vi "pdv_usb1.vi"() -> ()   [LabVIEW 2010]
uses:
  70user.lib/TheSigTab.vi
  <vilib>/Utility/config.llb/Read Key (U32).vi
  <vilib>/addons/database/Connection.llb/DB Tools Open Connec (Path).vi
  <vilib>/Utility/config.llb/Read Key (String).vi
  <vilib>/Utility/config.llb/Write Key (Double).vi
  <vilib>/Utility/config.llb/Write Key (U32).vi
  <vilib>/addons/database/NI_Database_API.lvlib
  <vilib>/Utility/config.llb/NI_LVConfig.lvlib
panel:
  in  "ScopeToo":bool caption="Сохранять осциллограммы"
  in  "m_s":u16(ring) items=["мин", "сек"]
  in  "Object":string(combo) caption="Объект"
  in  "CurvesToo":bool caption="Сохранять графики"
  in  "AcqureTime":dbl caption="опроса" format="%#.3g"
  out "ExtDev":bool caption="Выносной модуль"
  in  "SaveTime":dbl=1.0 caption="мин" min=1.0 max=120.0
  out "Slide":u8(slide) scale=0.0..100.0
  in  "Continuosly":bool caption="Периодически"
  in  "SaveNow":bool caption="Однократно"
  in  "Loop":bool caption="Зациклить данные"
  out "Current time":timestamp caption="Время и Дата" format="%<%X\n%x>T"
  out "Tper":dbl caption="общая"
  in  "filter":bool caption="Фильтр\nперекрёстных помех"
  in  "Stop":bool
  in  "Table":string[][](table) caption="Результаты измерений"
  # "Запись в базу данных"
  # "Продолжительность, с"
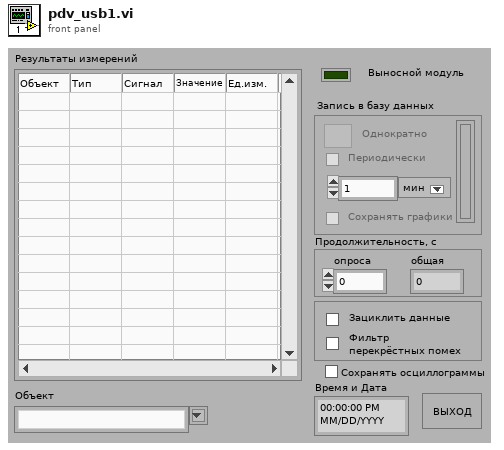
[diagram p1: front panel]
types:
  T1 = typedef "NI_LVConfig.lvlib/Config Data RefNum.ctl" = refnum<k1>
  T2 = typedef "NI_Database_API.lvlib/Conn ObjectReference.ctl" = refnum<k1>
  T3 = cluster{"Status":bool, "ViErrorNumber":u32, "ViName":string, "ViErrorString":string, "CinName":string, "CinErrorString":string}
  T4 = cluster{"VirtualSlot":u16, "ModuleName":string, "SerialNumber":string, "UsbSpeed":u8, "AvrVersion":string, "ModuleRevision":string, "DspType":string, "IsDacPresented":bool, "DspLoading":bool, "DspVersion":string, "DspClockout":u32, "AdcOffsetCoef":sgl[], "AdcScaleCoef":sgl[], "DacOffsetCoef":sgl[], "DacScaleCoef":sgl[]}
  T5 = cluster{"DllVersion":u32, "InterfaceType":u32, "InterfaceInstance":u32, "ModuleHandle":u32, "ReadBuffersParsArray":cluster{"Buffer":i16[], "ReadOv":u32, "ReadEvent":u32}[], "WriteBuffersParsArray":cluster{"Buffer":i16[], "WriteOv":u32, "WriteEvent":u32}[]}
  T6 = cluster{"Сигнал":string, "Тип":enum16{"Напряжение/Ток", "ЧР", "Температура", "Давление"}, "Object":string}[]
  T7 = cluster{"Сигнал":string, "Тип":enum16{"Напряжение/Ток", "ЧР", "Температура", "Давление"}, "Object":string}
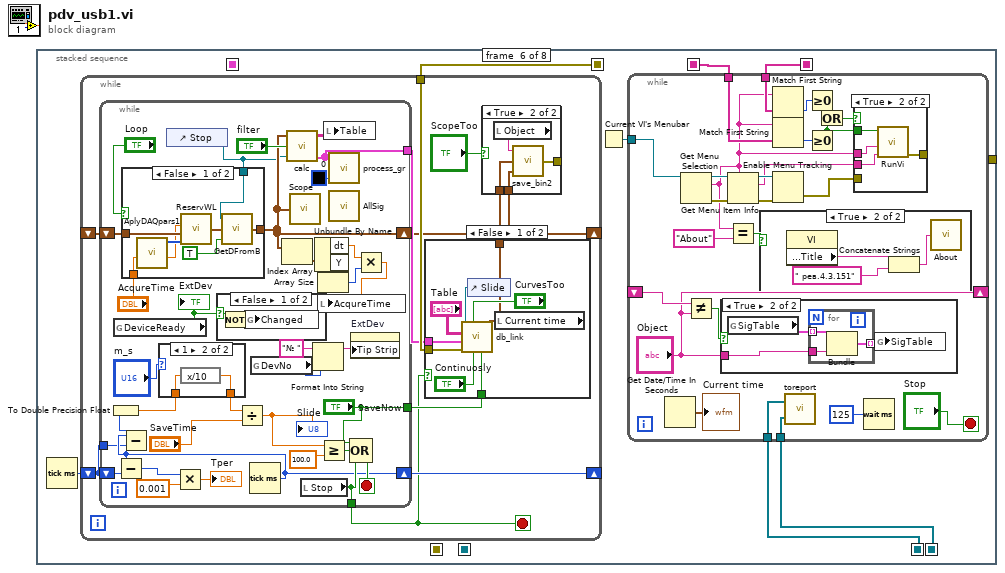
[diagram p0: block diagram]
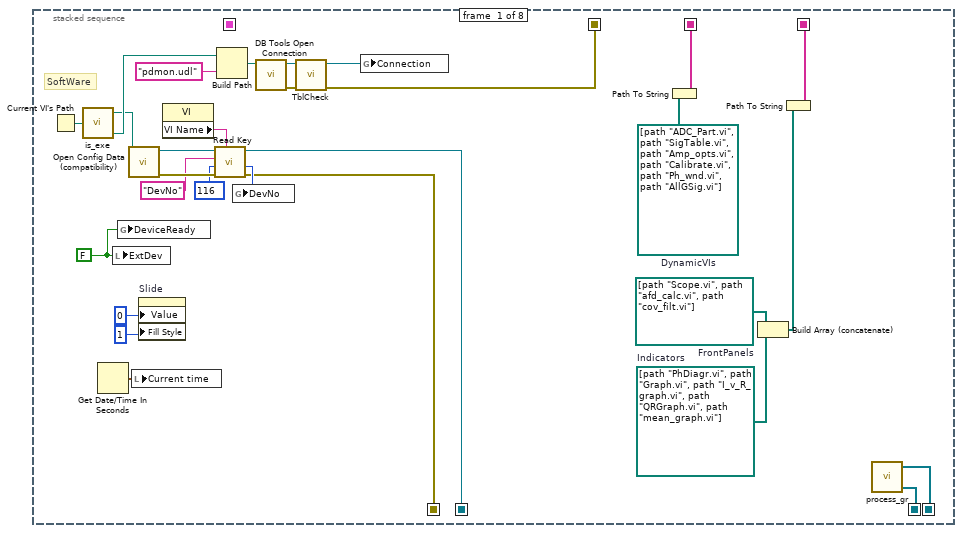
[diagram p2: hidden frame]
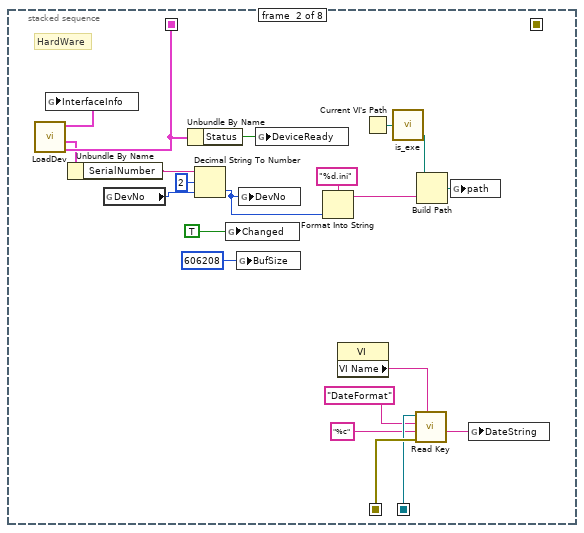
[diagram p3: hidden frame]
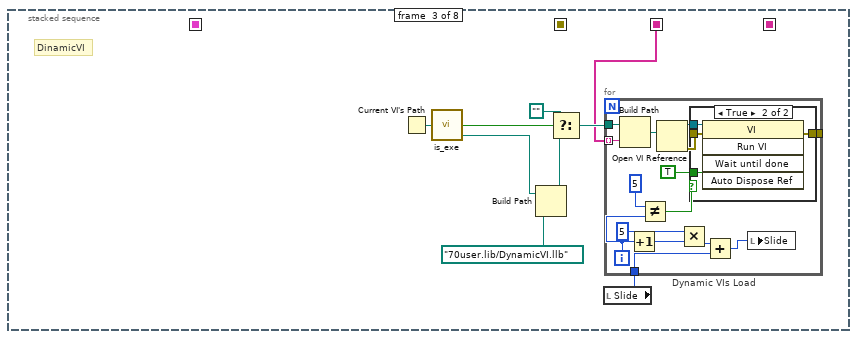
[diagram p4: hidden frame]
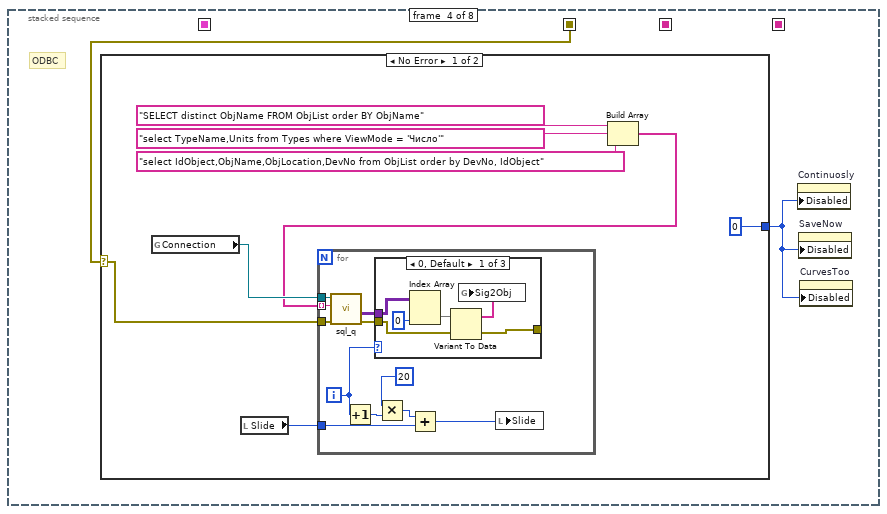
[diagram p6: hidden frame]
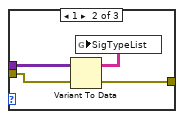
[diagram p7: hidden frame]
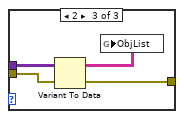
[diagram p8: hidden frame]
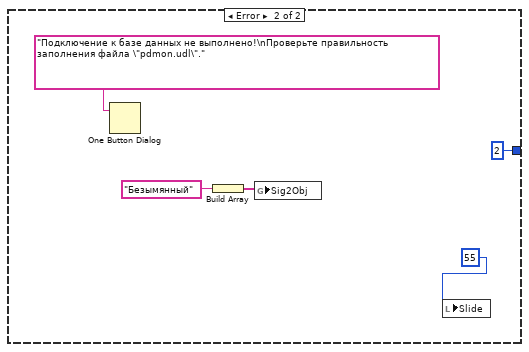
[diagram p9: hidden frame]
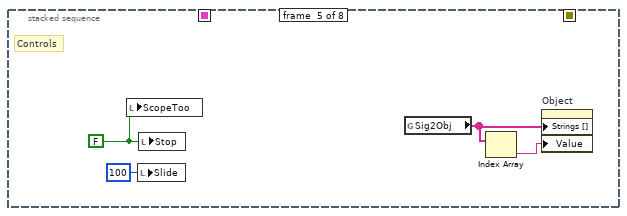
[diagram p10: hidden frame]
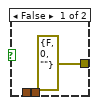
[diagram p11: hidden frame]
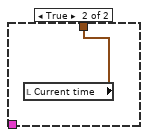
[diagram p12: hidden frame]
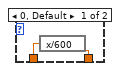
[diagram p13: hidden frame]
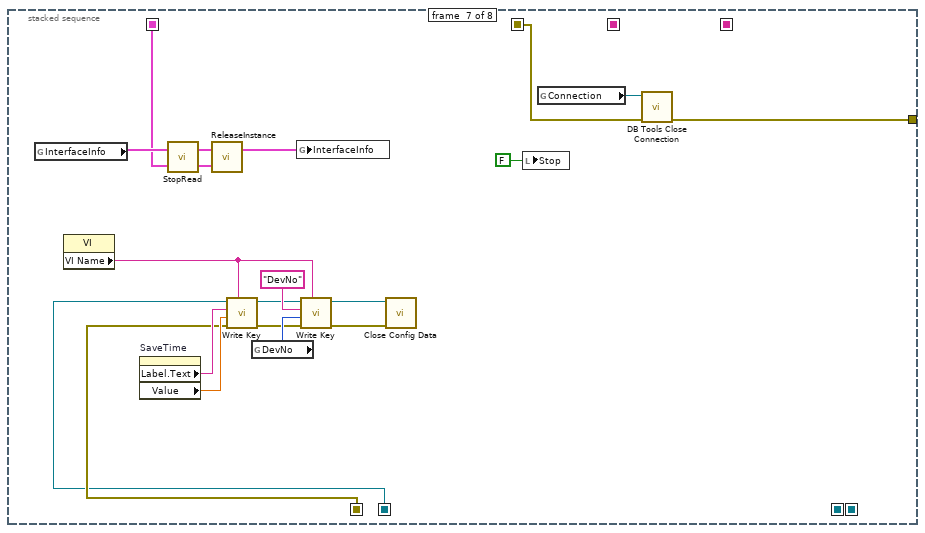
[diagram p19: hidden frame]
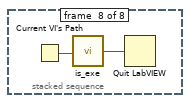
[diagram p20: hidden frame]
diagram:
  n1 = stacked-sequence {
    seq-local: [_ w45 _ _ _ _ _ _] -> [_ _ _ _ _ _ w256 _]
    seq-local: [w15 _ _ _ _ _ _ _] -> [_ _ _ w81 _ w129 w263 _]
    seq-local: [w18 _ _ _ _ _ _ _] -> [_ _ _ _ _ w127 _ _]
    seq-local: [w22 _ _ _ _ _ _ _] -> [_ _ w54 _ _ w126 _ _]
    seq-local: [w25 _ _ _ _ _ _ _] -> [_ _ _ _ _ w124 _ _]
    seq-local: [w24 _ _ _ _ _ _ _] -> [_ _ _ _ _ w125 _ _]
    seq-local: [w2 _ _ _ _ _ _ _] -> [_ w34 _ _ _ _ w244 _]
    seq-local: [w1 _ _ _ _ _ _ _] -> [_ w35 _ _ _ _ w245 _]
    tunnel: [_ _ _ _ _ _ w260 _] -> _
    frame #0 {
      w4 = FALSE ("ExtDev")
      w20 = path[] [path "PhDiagr.vi", path "Graph.vi", path "I_v_R_graph.vi", path "QRGraph.vi", path "mean_graph.vi"]  # Indicators
      w21 = path[] [path "Scope.vi", path "afd_calc.vi", path "cov_filt.vi"]  # FrontPanels
      w23 = path[] [path "ADC_Part.vi", path "SigTable.vi", path "Amp_opts.vi", path "Calibrate.vi", path "Ph_wnd.vi", path "AllGSig.vi"]  # DynamicVIs
      # "SoftWare"
      n2 = Current VI's Path() -> (path=w29:path)
      n3 = call "is_exe.vi"("path"=w29) -> ("actual path"=w28:path, "ini path"=w10:path)  [unwired: 2 in, 1 out]
      n4 = Get Date/Time In Seconds() -> (seconds since 1Jan1904=w13:timestamp)
      n5 = local write "ExtDev"(w4) -> ()
      n6 = global write "TheSigTab.vi" "DeviceReady"(w4) -> ()
      n7 = call <vilib>:"Open Config Data (compatibility).vi"("configuration file path"=w10) -> ("error out"=w8:errorcluster, "refnum"=w9:T1)  [unwired: 8 in, 1 out]
      n8 = local write "Current time"(w13) -> ()
      n9 = property on="Slide" class="Slide (strict)"("Value"=u8 0 ("Slide"), "Fill Style"=1) -> ()  [unwired: 2 in, 2 out]
      n10 = property class="VI"() -> ("VI Name"=w3:string)  [unwired: 2 in, 2 out]
      n11 = call-poly <vilib>:"Read Key.vi"("section"=w3, "error in (no error)"=w8, "default value"=u32 116 ("DevNo"), "key"="DevNo", "refnum"=w9) -> ("error out"=w1:errorcluster, "value"=w5:u32, "refnum out"=w2:T1)  [unwired: 3 in, 1 out]
      n12 = Build Path(base path=w28, name or relative path="pdmon.udl") -> (appended path=w26:path)
      n13 = global write "TheSigTab.vi" "DevNo"(w5) -> ()
      n14 = call-poly <vilib>:"DB Tools Open Connection.vi"("connection information"=w26) -> ("error out"=w16:errorcluster, "connection reference"=w17:T2)  [unwired: 7 in]
      n15 = call "TblCheck.vi"("error in"=w16, "connection reference"=w17) -> ("error out"=w15:errorcluster, "conn ref out"=w14:T2)  [unwired: 3 in, 1 out]
      n16 = global write "TheSigTab.vi" "Connection"(w14) -> ()
      n17 = Path To String(path=w23) -> (string=w22:string[])
      n18 = Build Array (concatenate)(w21, w20) -> (w19:path[])
      n19 = Path To String(path=w19) -> (string=w18:string[])
      n20 = call "process_gr.vi"() -> ("WG refs"=w25:refnum<vi>[], "menu refs"=w24:refnum<k9>[])  [unwired: 4 in]
    }
    frame #1 {
      # "HardWare"
      n21 = call "LoadDev.vi"() -> ("ViStatus"=w45:T3, "ModuleInfo"=w44:T4, "InterfaceInfo"=w46:T5)  [unwired: 5 in]
      n22 = global write "TheSigTab.vi" "InterfaceInfo"(w46) -> ()
      n23 = Unbundle By Name(w44) -> ("SerialNumber"=w43:string)
      n24 = global read "TheSigTab.vi" "DevNo"() -> (w36:u32)
      n25 = Unbundle By Name(w45) -> ("Status"=w50:bool)
      n26 = Decimal String To Number(string=w43, offset=u32 2 ("initial scan location"), default (0L)=w36) -> (number=w38:u32)  [unwired: 1 out]
      n27 = global write "TheSigTab.vi" "Changed"(TRUE ("Changed")) -> ()
      n28 = global write "TheSigTab.vi" "BufSize"(u32 606208 ("BufSize")) -> ()
      n29 = global write "TheSigTab.vi" "DevNo"(w38) -> ()
      n30 = global write "TheSigTab.vi" "DeviceReady"(w50) -> ()
      n31 = Format Into String(format string="%d.ini", w38) -> (resulting string=w40:string)  [unwired: 2 in, 1 out]
      n32 = property class="VI"() -> ("VI Name"=w33:string)  [unwired: 2 in, 2 out]
      n33 = Current VI's Path() -> (path=w49:path)
      n34 = call "is_exe.vi"("path"=w49) -> ("actual path"=w37:path)  [unwired: 2 in, 2 out]
      n35 = call-poly <vilib>:"Read Key.vi"("section"=w33, "error in (no error)"=w35, "default value"="%c", "key"="DateFormat", "refnum"=w34) -> ("value"=w30:string)  [unwired: 3 in, 3 out]
      n36 = Build Path(base path=w37, name or relative path=w40) -> (appended path=w39:path)
      n37 = global write "TheSigTab.vi" "path"(w39) -> ()
      n38 = global write "TheSigTab.vi" "DateString"(w30) -> ()
    }
    frame #2 {
      # "DinamicVI"
      n39 = Current VI's Path() -> (path=w53:path)
      n40 = call "is_exe.vi"("path"=w53) -> ("actual path"=w51:path, "exe?"=w52:bool)  [unwired: 2 in, 1 out]
      n41 = Build Path(base path=w51, name or relative path=path "70user.lib/DynamicVI.llb" ("f")) -> (appended path=w55:path)
      n42 = Select(t=path "", s=w52, f=w55) -> (s? t:f=w59:path)
      n43 = local read "Slide"() -> (w58:u8)
      n44 = for "Dynamic VIs Load" {
        tunnel: w54 -> [w74] mode=indexing
        tunnel: w59 -> [w72]
        tunnel: w58 -> [w68]
        tunnel: [w63] -> _
        i -> [w62]
        n45 = Build Path(base path=w72, name or relative path=w74) -> (appended path=w73:path)
        n46 = Increment(x=w62) -> (x+1=w64:i32)
        n47 = Not Equal?(x=5, y=w62) -> (x != y?=w60:bool)
        n48 = Open VI Reference(vi path=w73) -> (vi reference=w70:refnum<vi>, error out=w69:errorcluster)  [unwired: 5 in]
        n49 = Multiply(x=5, y=w64) -> (x*y=w66:i32)
        n50 = case shown="True" w60 {
          tunnel: TRUE ("Wait until done") -> [_ w79]
          tunnel: w70 -> [_ w78]
          tunnel: w69 -> [w75 w77]
          tunnel: [w75 w76] -> w63
          frame False {
          }
          frame True {
            n51 = invoke class="VI" method="Run VI"(reference=w78, error in=w77, "Wait until done"=w79) -> (error out=w76:errorcluster)  [unwired: 2 in, 4 out]
          }
        }
        n52 = Add(x=w66, y=w68) -> (x+y=w67:i32)
        n53 = local write "Slide"(w67) -> ()
      }
    }
    frame #3 {
      # "ODBC"
      n54 = case shown="No Error" w81 {
        selector: w81 -> [w85 _]
        tunnel: [u8 0 ("Disabled") u8 2 ("Disabled")] -> w80
        frame No Error {
          n55 = global read "TheSigTab.vi" "Connection"() -> (w86:T2)
          n56 = local read "Slide"() -> (w83:u8)
          n57 = Build Array("SELECT distinct ObjName FROM ObjList order BY ObjName", "select TypeName,Units from Types where ViewMode = 'Число'", "select IdObject,ObjName,ObjLocation,DevNo from ObjList order by DevNo, IdObject" ("table")) -> (w84:string[])
          n58 = for {
            tunnel: w86 -> [w99]
            tunnel: w85 -> [w98]
            tunnel: w84 -> [w96] mode=indexing
            tunnel: w83 -> [w95]
            i -> [w92]
            n59 = call "sql_q.vi"("error in"=w98, "SQL query"=w96, "connect ref"=w99) -> ("error out"=w97:errorcluster, "recordset data"=w100:variant[][])  [unwired: 1 in, 2 out]
            n60 = Increment(x=w92) -> (x+1=w90:i32)
            n61 = case shown="0, Default" w92 {
              tunnel: w100 -> [w103 w110 w114]
              tunnel: w97 -> [w102 w108 w112]
              tunnel: [w101 w107 w111] -> _
              frame 0, Default {
                n62 = Index Array(array=w103, index (col)=0 ("disabled index (col)")) -> (element=w105:variant[])  [unwired: 1 in]
                n63 = Variant To Data(error in=w102, Variant=w105) -> (error out=w101:errorcluster, data=w104:string[])  [unwired: 1 in]
                n64 = global write "TheSigTab.vi" "Sig2Obj"(w104) -> ()
              }
              frame 1 {
                n65 = Variant To Data(error in=w108, Variant=w110) -> (error out=w107:errorcluster, data=w109:string[][])  [unwired: 1 in]
                n66 = global write "TheSigTab.vi" "SigTypeList"(w109) -> ()
              }
              frame 2 {
                n67 = Variant To Data(error in=w112, Variant=w114) -> (error out=w111:errorcluster, data=w113:string[][])  [unwired: 1 in]
                n68 = global write "TheSigTab.vi" "ObjList"(w113) -> ()
              }
            }
            n69 = Multiply(x=20, y=w90) -> (x*y=w93:i32)
            n70 = Add(x=w93, y=w95) -> (x+y=w94:i32)
            n71 = local write "Slide"(w94) -> ()
          }
        }
        frame Error {
          n72 = One Button Dialog(message="Подключение к базе данных не выполнено!\nПроверьте правильность заполнения файла \"pdmon.udl\".") -> ()  [unwired: 1 in, 1 out]
          n73 = Build Array("Безымянный" ("table")) -> (w118:string[])
          n74 = global write "TheSigTab.vi" "Sig2Obj"(w118) -> ()
          n75 = local write "Slide"(u8 55 ("Slide")) -> ()
        }
      }
      n76 = property on="Continuosly" class="Bool (strict)"("Disabled"=w80) -> ()  [unwired: 2 in, 2 out]
      n77 = property on="SaveNow" class="Bool"("Disabled"=w80) -> ()  [unwired: 2 in, 2 out]
      n78 = property on="CurvesToo" class="Bool (strict)"("Disabled"=w80) -> ()  [unwired: 2 in, 2 out]
    }
    frame #4 {
      w120 = FALSE ("Changed")
      # "Controls"
      n79 = local write "ScopeToo"(w120) -> ()
      n80 = local write "Slide"(u8 100 ("Slide")) -> ()
      n81 = local write "Stop"(w120) -> ()
      n82 = global read "TheSigTab.vi" "Sig2Obj"() -> (w122:string[])
      n83 = Index Array(array=w122) -> (element=w121:string)  [unwired: 1 in]
      n84 = property on="Object" class="CmbBox"("Strings []"=w122, "Value"=w121) -> ()  [unwired: 2 in, 2 out]
    }
    frame #5 {
      n85 = Tick Count (ms)() -> (millisecond timer value=w130:u32)
      n86 = while {
        shift-right: [w140] -> _
        shift-left: w130 -> [w137]
        shift-right: [w133] -> _
        shift-left: _ -> [w139]
        tunnel: w129 -> [w138]
        stop <- w134 stop-if-true
        n87 = while {
          shift-right: [w167] -> w133
          shift-left: w139 -> [w186]
          shift-right: [w181] -> w140
          shift-left: w137 -> [w187]
          tunnel: [w183] -> w134
          tunnel: w137 -> [w180]
          tunnel: ["SaveNow"] -> w136
          tunnel: [w173] -> w135
          stop <- w182 stop-if-true
          n88 = global read "TheSigTab.vi" "DeviceReady"() -> (w178:bool)
          "ExtDev" <- w178
          n89 = control-ref of="Stop"() -> (w161:refnum<vi>)
          n90 = case shown="False" "Loop" {
            tunnel: w186 -> [w203 w204]
            tunnel: [w200 w204] -> w167
            tunnel: "AcqureTime" -> [w197 _]
            tunnel: w161 -> [w196 _]
            frame False {
              n91 = call "AplyDAQpars1.vi"("AcqTimeIn"=w197) -> ("t1-t0"=w198:dbl, "Idxs"=w202:i32[])  [unwired: 5 in]
              n92 = call "ReservWL.vi"("Tags"=w202, "ArrayIn"=w203, "t1-t0"=w198) -> ("Array"=w201:waveform(i16)[])  [unwired: 1 in]
              n93 = call "GetDFromB.vi"("Control"=TRUE, "ArrayIn"=w201, "Bool Refnum"=w196) -> ("ArrayOut"=w200:waveform(i16)[])
            }
            frame True {
            }
          }
          n94 = case shown="False" w178 {
            selector: w178 -> [w195 _]
            frame False {
              n95 = Not(x=w195) -> (.not. x?=w194:bool)
              n96 = global write "TheSigTab.vi" "Changed"(w194) -> ()
            }
            frame True {
            }
          }
          n97 = Tick Count (ms)() -> (millisecond timer value=w181:u32)
          n98 = Subtract(x=w181, y=w187) -> (x-y=w177:u32)
          n99 = Subtract(x=w181, y=w180) -> (x-y=w179:u32)
          n100 = To Double Precision Float(number=w179) -> (double precision float=w156:dbl)
          n101 = case shown="1" "m_s" {
            tunnel: w156 -> [w191 w193]
            tunnel: [w190 w192] -> w155
            frame 0, Default {
              n102 = expression code="x/600"(w191) -> (w190:dbl)
            }
            frame 1 {
              n103 = expression code="x/10"(w193) -> (w192:dbl)
            }
          }
          n104 = Multiply(x=w177, y=0.001 ("x")) -> (x*y=→"Tper":dbl)
          n105 = Divide(x=w155, y="SaveTime") -> (x/y=w171:dbl)
          "Slide" <- w171
          n106 = global read "TheSigTab.vi" "DevNo"() -> (w158:u32)
          n107 = Index Array(array=w167) -> (element=w166:waveform(i16))  [unwired: 1 in]
          n108 = call "calc.vi"("Acquire"=w161, "filter"="filter", "ArrayIn"=w167) -> ("AllMeasures"=w173:cluster{"x0":dbl, "dx":dbl, "y":sgl[][]}[], "Values"=w189:string[][])  [unwired: 1 in]
          n109 = call "Scope.vi"("Array"=w167) -> ()
          n110 = local read "Stop"() -> (w183:bool)
          n111 = Format Into String(initial string="№ ", w158) -> (resulting string=w160:string)  [unwired: 2 in, 1 out]
          n112 = Unbundle By Name(w166) -> ("dt"=w164:dbl, "Y"=w165:i16[])
          n113 = Array Size(array=w165) -> (size(s)=w163:i32)
          n114 = Greater Or Equal?(x=w171, y=100.0 ("x")) -> (x >= y?=w168:bool)
          n115 = local write "Table"(w189) -> ()
          n116 = call "process_gr.vi"("Color Box"=u32 0, "AllMeasures"=w173) -> ()  [unwired: 2 in, 2 out]
          n117 = call "AllSig.vi"() -> ()  [unwired: 1 in]
          n118 = Compound Arithmetic op=OR("SaveNow", w168, w183) -> (w182:bool)
          n119 = property on="ExtDev" class="Bool (strict)"("Tip Strip"=w160) -> ()  [unwired: 2 in, 2 out]
          n120 = Multiply(x=w164, y=w163) -> (x*y=w162:dbl)
          n121 = local write "AcqureTime"(w162) -> ()
        }
        n122 = case shown="False" w134 {
          tunnel: w138 -> [w153 _]
          tunnel: w136 -> [w152 _]
          tunnel: w135 -> [w150 _]
          tunnel: [w146 w154] -> w132
          frame False {
            n123 = control-ref of="Slide"() -> (w149:refnum<vi>)
            n124 = local read "Current time"() -> (w146:timestamp)
            n125 = call "db_link.vi"("Current time"=w146, "SaveNow"=w152, "Continuosly"="Continuosly", "SaveCurves?"="CurvesToo", "error in"=w153, "AllMeasures"=w150, "Table"="Table", "reference"=w149) -> ()  [unwired: 3 in, 1 out]
          }
          frame True {
            n126 = local read "Current time"() -> (w154:timestamp)
          }
        }
        n127 = case shown="True" "ScopeToo" {
          tunnel: [errorcluster {"status"=FALSE, "code"=0, "source"=""} ("error out") w145] -> _
          tunnel: w133 -> [_ w144]
          tunnel: w132 -> [_ w143]
          frame False {
          }
          frame True {
            n128 = local read "Object"() -> (w142:string)
            n129 = call "save_bin2.vi"("ArrayOut"=w144, "Current time"=w143, "Object"=w142) -> ("error out"=w145:errorcluster)
          }
        }
      }
      n130 = Current VI's Menubar() -> (w128:refnum<k9>)
      n131 = while {
        tunnel: w128 -> [w226]
        tunnel: w127 -> [w222]
        tunnel: w126 -> [w219]
        tunnel: w125 -> [w217]
        tunnel: w124 -> [w216]
        shift-right: ["Object"] -> _
        shift-left: _ -> [w209]
        stop <- "Stop" stop-if-true
        n132 = Get Date/Time In Seconds() -> (seconds since 1Jan1904=→"Current time":timestamp)
        n133 = Get Menu Selection(0:w226) -> (5:w225:refnum<k9>, 6:w207:string, 8:w218:errorcluster)  [unwired: 3 in, 2 out]
        n134 = Not Equal?(x=w209, y="Object") -> (x != y?=w210:bool)
        n135 = case shown="True" w210 {
          tunnel: "Object" -> [_ w233]
          frame False {
          }
          frame True {
            n136 = global read "TheSigTab.vi" "SigTable"() -> (w235:T6)
            n137 = for {
              tunnel: w235 -> [w238] mode=indexing
              tunnel: w233 -> [w237]
              tunnel: [w236] -> w234 mode=indexing
              n138 = Bundle(cluster=w238, "Object"=w237) -> (w236:T7)  [unwired: 2 in]
            }
            n139 = global write "TheSigTab.vi" "SigTable"(w234) -> ()
          }
        }
        n140 = Get Menu Item Info(7:w207, 8:w218, 11:w225) -> (0:w215:errorcluster, 2:w221:string, 3:w224:refnum<k9>)  [unwired: 4 out]
        n141 = Equal?(x=w207, y="About") -> (x = y?=w205:bool)
        n142 = case shown="True" w205 {
          frame False {
          }
          frame True {
            n143 = property class="VI"() -> ("Front Panel Window:Title"=w232:string)  [unwired: 2 in, 2 out]
            n144 = Concatenate Strings(w232, " рев.4.3.151" ("input 1")) -> (w230:string)
            n145 = call "About.vi"("Revision Number"=w230) -> ()
          }
        }
        n146 = Match First String(2:w222, 3:w207) -> (0:w223:i32)  [unwired: 1 out]
        n147 = Match First String(2:w219, 3:w207) -> (0:w220:i32)  [unwired: 1 out]
        n148 = Enable Menu Tracking(2:w215, 4:w224) -> (0:w211:errorcluster)  [unwired: 1 in, 1 out]
        n149 = call "toreport.vi"("Menu"=w217, "WG"=w216) -> ()
        n150 = Greater Or Equal To 0?(x=w223) -> (x >= 0?=w214:bool)
        n151 = Greater Or Equal To 0?(x=w220) -> (x >= 0?=w213:bool)
        n152 = Or(x=w214, y=w213) -> (x .or. y?=w212:bool)
        n153 = case shown="True" w212 {
          tunnel: w221 -> [_ w243]
          tunnel: w207 -> [_ w242]
          tunnel: w213 -> [_ w241]
          tunnel: w211 -> [w239 _]
          tunnel: [w239 w240] -> _
          frame False {
          }
          frame True {
            n154 = call "RunVi.vi"("Title"=w243, "Name"=w242, "Run/JustOpen"=w241) -> ("error out"=w240:errorcluster)  [unwired: 4 in]
          }
        }
        n155 = Wait (ms)(milliseconds to wait=u32 125) -> ()  [unwired: 1 out]
      }
    }
    frame #6 {
      n156 = global read "TheSigTab.vi" "InterfaceInfo"() -> (w258:T5)
      n157 = property class="VI"() -> ("VI Name"=w250:string)  [unwired: 2 in, 2 out]
      n158 = property on="SaveTime" class="DigNum (strict)"() -> ("Label.Text"=w247:string, "Value"=w246:dbl)  [unwired: 2 in, 2 out]
      n159 = call "StopRead.vi"("ViStatusIn"=w256, "InterfaceInfoIn"=w258) -> ("ViStatusOut"=w255:T3, "InterfaceInfoOut"=w257:T5)
      n160 = call "ReleaseInstance.vi"("ViStatusIn"=w255, "InterfaceInfoIn"=w257) -> ("InterfaceInfoOut"=w259:T5)  [unwired: 1 out]
      n161 = call-poly <vilib>:"Write Key.vi"("section"=w250, "error in (no error)"=w245, "value"=w246, "key"=w247, "refnum"=w244) -> ("error out"=w248:errorcluster, "refnum out"=w249:T1)  [unwired: 4 in, 1 out]
      n162 = global read "TheSigTab.vi" "DevNo"() -> (w252:u32)
      n163 = global write "TheSigTab.vi" "InterfaceInfo"(w259) -> ()
      n164 = call-poly <vilib>:"Write Key.vi"("section"=w250, "error in (no error)"=w248, "value"=w252, "key"="DevNo", "refnum"=w249) -> ("error out"=w253:errorcluster, "refnum out"=w254:T1)  [unwired: 4 in, 1 out]
      n165 = call <vilib>:"Close Config Data.vi"("error in (no error)"=w253, "refnum"=w254) -> ()  [unwired: 8 in, 2 out]
      n166 = local write "Stop"(FALSE ("Stop")) -> ()
      n167 = global read "TheSigTab.vi" "Connection"() -> (w262:T2)
      n168 = call <vilib>:"DB Tools Close Connection.vi"("error in (no error)"=w263, "connection reference"=w262) -> ("error out"=w260:errorcluster)  [unwired: 5 in]
    }
    frame #7 {
      n169 = Current VI's Path() -> (path=w264:path)
      n170 = call "is_exe.vi"("path"=w264) -> ("exe?"=w265:bool)  [unwired: 2 in, 2 out]
      n171 = Quit LabVIEW(quit? (T)=w265) -> ()
    }
  }
